vi "To String Array.vi"(8 "error in (no error)":errorcluster, 11 "Wait On Integer Step Config in":refnum<class "Wait On Integer Config.lvclass">) -> (0 "error out":errorcluster, 1 "Step String Array":string[](array[string]), 3 "Wait On Integer Step Config out":refnum<class "Wait On Integer Config.lvclass">)   [LabVIEW 2015, in "Wait On Integer Config.lvclass"]
uses:
  Wait On Integer Config.lvclass
  Wait On Integer Config.lvclass/Wait On Integer Config.ctl
  <vilib>/NI/Tag Bus/tag/tag descriptor.lvclass/tag descriptor.ctl
  classes/Step/Config/Step Config.lvclass
  <vilib>/NI/Tag Bus/tag/tag descriptor.lvclass
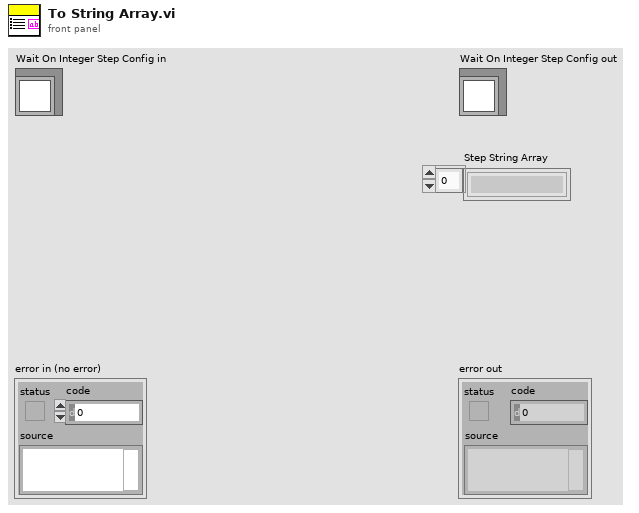
[diagram p1: front panel]
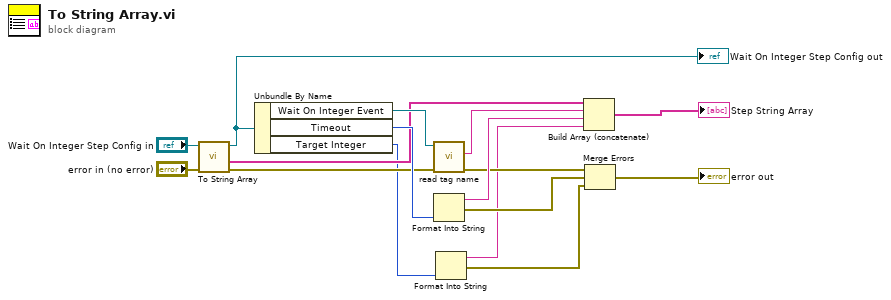
[diagram p0: block diagram]
diagram:
  n1 = call-parent "To String Array.vi"("error in (no error)"="error in (no error)", "Step Config in"="Wait On Integer Step Config in") -> ("error out"=w12:errorcluster, "Step String Array"=w10:string[], "Step Config out"=w11:refnum<class "Wait On Integer Config.lvclass">)  [unwired: 7 in]
  "Wait On Integer Step Config out" <- w11
  n2 = Unbundle By Name(w11) -> ("Wait On Integer Event"=w13:refnum<class "TBM channel.lvclass">, "Timeout"=w14:i32, "Target Integer"=w3:u32)
  n3 = call <vilib>:"read tag name.vi"("error in"=w12, "system tag in"=w13) -> ("error out"=w5:errorcluster, "name"=w9:string)  [unwired: 7 in, 1 out]
  n4 = Format Into String(w14) -> (resulting string=w8:string, error out=w6:errorcluster)  [unwired: 3 in]
  n5 = Format Into String(w3) -> (resulting string=w1:string, error out=w2:errorcluster)  [unwired: 3 in]
  n6 = Build Array (concatenate)(w10, w9, w8, w1) -> (→"Step String Array":string[])
  n7 = Merge Errors(w5, w6, w2) -> (→"error out":errorcluster)
